vi "Scale Remote Coordinates to Servo Values.vi"(2 "Low Range":i32, 3 "Remote Input":i32, 4 "High Range":i32) -> (0 "Output":i32)   [LabVIEW 2010, in "Tetrix.lvlib"]
uses:
  Tetrix.lvlib
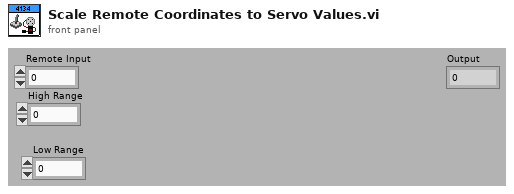
[diagram p1: front panel]
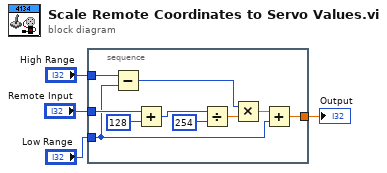
[diagram p0: block diagram]
diagram:
  n1 = stacked-sequence {
    tunnel: "Remote Input" -> [w14]
    tunnel: "High Range" -> [w10]
    tunnel: "Low Range" -> [w6]
    tunnel: [w5] -> w1
    frame #0 {
      n2 = Subtract(x=w10, y=w6) -> (x-y=w9:i32)
      n3 = Add(x=w14, y=128) -> (x+y=w12:i32)
      n4 = Divide(x=w12, y=254) -> (x/y=w8:dbl)
      n5 = Multiply(x=w9, y=w8) -> (x*y=w7:dbl)
      n6 = Add(x=w7, y=w6) -> (x+y=w5:dbl)
    }
  }
  "Output" <- w1
